vi "Create.vi"(8 "error in (no error)":errorcluster, 9 "settings":T1, 10 "Transfer Groups Configurations":T2[](array[typedef]) {"Transfers"."channels"."dst buffer offset" format="%d bytes"; "Transfers"."channels"."src buffer offset" format="%d bytes"}, 11 "Buffer Converter type":refnum<class "Buffer Converter.lvclass">) -> (0 "error out":errorcluster, 3 "Buffer Converter out":refnum<class "Buffer Converter.lvclass">)   [LabVIEW 2017, in "DSF Core.lvlib" / "Buffer Converter.lvclass"]
uses:
  Buffer Converter.lvclass
  DSF Configuration API/Public/Controls/DSF Engine Transfer Group Configuration.ctl
  DSF Configuration API/Public/Controls/DSF Direction.ctl
  DSF Configuration API/Public/Controls/DSF Timing Info.ctl
  DSF Configuration API/Public/Controls/DSF Engine Transfer Configuration.ctl
  DSF Configuration API/Public/Controls/DSF Byte Order.ctl
  DSF Configuration API/Public/Controls/DSF Engine Channel Configuration.ctl
  DSF Configuration API/Public/Controls/DSF Data Type.ctl
  DSF Configuration API/Public/Controls/DSF Settings Info.ctl
  DSF Core.lvlib
  DSF Configuration API/Public/Largest Contiguous Channel Count (Transfer Group).vi
  DSF Configuration API/Public/Max Block Count (Transfer Group).vi
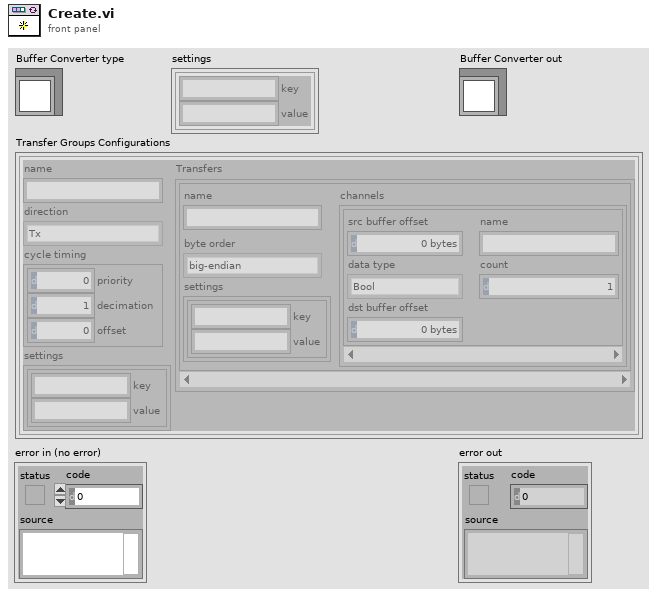
[diagram p1: front panel]
types:
  T1 = typedef "DSF Core.lvlib/DSF Settings Info.ctl" = cluster{"key":string, "value":string}[]
  T2 = typedef "DSF Core.lvlib/DSF Engine Transfer Group Configuration.ctl" = cluster{"name":string, "direction":T3, "cycle timing":T4, "Transfers":T5[], "settings":T1}
  T3 = typedef "DSF Core.lvlib/DSF Direction.ctl" = enum8{"Tx", "Rx"}
  T4 = typedef "DSF Core.lvlib/DSF Timing Info.ctl" = cluster{"priority":u64, "decimation":u64, "offset":u64}
  T5 = typedef "DSF Core.lvlib/DSF Engine Transfer Configuration.ctl" = cluster{"name":string, "byte order":T6, "channels":T7[], "settings":T1}
  T6 = typedef "DSF Core.lvlib/DSF Byte Order.ctl" = enum8{"big-endian", "little-endian"}
  T7 = typedef "DSF Core.lvlib/DSF Engine Channel Configuration.ctl" = cluster{"src buffer offset":u64, "name":string, "data type":T8, "count":u64, "dst buffer offset":u64}
  T8 = typedef "DSF Core.lvlib/DSF Data Type.ctl" = enum8{"Bool", "SGL", "DBL", "I8", "I16", "I32", "I64", "U8", "U16", "U32", "U64"}
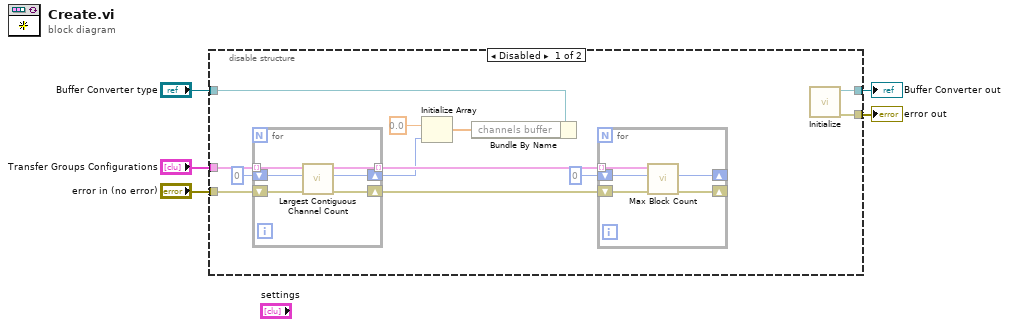
[diagram p0: block diagram]
diagram:
  n1 = disable-structure shown="Disabled" {
    disable-tunnel: "error in (no error)" -> [w16 w32]
    disable-tunnel: "Buffer Converter type" -> [w14 w33]
    disable-tunnel: [w8 w32] -> w3
    disable-tunnel: [w7 w33] -> w2
    disable-tunnel: "Transfer Groups Configurations" -> [w6 _]
    frame Disabled {
      n2 = for {
        tunnel: w6 -> [w23] mode=indexing
        shift-right: [w26] -> w11
        shift-left: u64 0 ("max channel count") -> [w21]
        shift-right: [w25] -> w18
        shift-left: w16 -> [w24]
        tunnel: [w22] -> w17 mode=indexing
        n3 = call-poly "Largest Contiguous Channel Count.vi"("error in (no error)"=w24, "largest contiguous channel count in (0)"=w21, "Transfer Group Configuration in"=w23) -> ("error out"=w25:errorcluster, "largest contiguous channel count out"=w26:u64, "Transfer Group Configuration out"=w22:T2)  [unwired: 6 in]
      }
      n4 = Initialize Array(0.0 ("element"), w11) -> (w10:dbl[])
      n5 = Bundle By Name(cluster=w14, "channels buffer"=w10) -> (w13:refnum<class "Buffer Converter.lvclass">)
      n6 = for {
        tunnel: w17 -> [w31] mode=indexing
        shift-right: [w27] -> w9
        shift-left: u64 0 ("max channel count") -> [w30]
        shift-right: [w28] -> w15
        shift-left: w18 -> [w29]
        n7 = call-poly "Max Block Count.vi"("error in (no error)"=w29, "largest block count in (0)"=w30, "Transfer Group in"=w31) -> ("error out"=w28:errorcluster, "largest block count out"=w27:u64)  [unwired: 6 in, 1 out]
      }
      n8 = call-dynamic "Initialize.vi"() -> ("error out"=w8:errorcluster, "Buffer Converter out"=w7:refnum<class "Buffer Converter.lvclass">)  [unwired: 10 in]
    }
    frame Enabled {
    }
  }
  "error out" <- w3
  "Buffer Converter out" <- w2
